vi "Set_Cells_pos.vi"(8 "error in (no error)":errorcluster, 10 "axis":i32, 11 "DelayLine in":refnum<class "DelayLine.lvclass">) -> (0 "error out":errorcluster, 3 "DelayLine out":refnum<class "DelayLine.lvclass">)   [LabVIEW 2020, in "DelayLine.lvclass"]
uses:
  DelayLine.lvclass
  C:/dev/TRANCON/Classes/GeneralFunctionality/GeneralFunctionality.lvclass
  GeneralFunctionality/GeneralFunctionality.lvclass/GeneralFunctionality.ctl
  DelayLine.lvclass/DelayLine.ctl
  Config/Config.lvclass
  GeneralFunctionality/GeneralFunctionality.lvclass
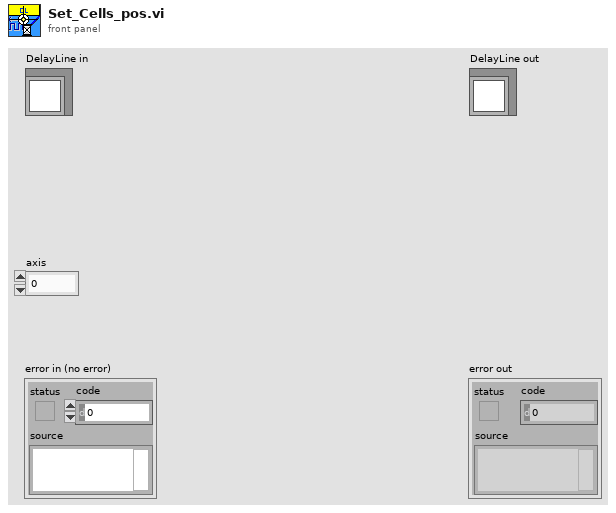
[diagram p1: front panel]
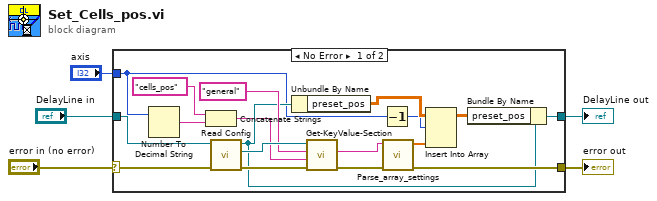
[diagram p0: block diagram]
diagram:
  n1 = case shown="No Error" "error in (no error)" {
    selector: "error in (no error)" -> [w22 w25]
    tunnel: [w17 w25] -> w4
    tunnel: [w15 w24] -> w2
    tunnel: "DelayLine in" -> [w23 w24]
    tunnel: "axis" -> [w7 _]
    frame No Error {
      n2 = Number To Decimal String(number=w7) -> (decimal integer string=w6:string)  [unwired: 1 in]
      n3 = Concatenate Strings("cells_pos" ("Key"), w6) -> (w8:string)
      n4 = call "Read Config.vi"("error in (no error)"=w22, "GeneralFunctionality en entrée"=w23) -> ("error out"=w21:errorcluster, "Config.lvclass"=w20:refnum<class "Config.lvclass">, "GeneralFunctionality en sortie"=w14:refnum<class "DelayLine.lvclass">)  [unwired: 7 in]
      n5 = Unbundle By Name(w14) -> ("preset_pos"=w13:dbl[][])
      n6 = call-dynamic "Get-KeyValue-Section.vi"("error in (no error)"=w21, "Key"=w8, "Section"="general", "Config in"=w20) -> ("error out"=w18:errorcluster, "Value"=w16:string)  [unwired: 5 in, 1 out]
      n7 = Decrement(x=w7) -> (x-1=w12:i32)
      n8 = call "Parse_array_settings.vi"("error in (no error)"=w18, "Value"=w16) -> ("error out"=w17:errorcluster, "Array"=w11:dbl[])  [unwired: 8 in]
      n9 = Insert Into Array(array=w13, index (row)=w12, new element=w11) -> (w10:dbl[][])  [unwired: 1 in]
      n10 = Bundle By Name(cluster=w14, "preset_pos"=w10) -> (w15:refnum<class "DelayLine.lvclass">)
    }
    frame Error {
    }
  }
  "error out" <- w4
  "DelayLine out" <- w2
